vi "button.vi"() -> ()   [LabVIEW 2023]
panel:
  out "Boolean":bool
  in  "OK Button 3":bool
  out "Boolean 3":bool
  in  "Boolean 2":bool
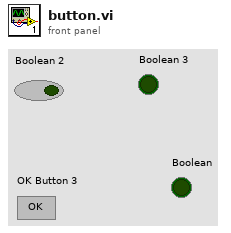
[diagram p1: front panel]
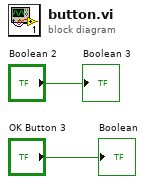
[diagram p0: block diagram]
diagram:
  "Boolean 3" <- "Boolean 2"
  "Boolean" <- "OK Button 3"
